vi "AndCriteria.vi"(8 "error in (no error)":errorcluster, 9 "Other Criteria":refnum<class "Criteria.lvclass">, 10 "Criteria":refnum<class "Criteria.lvclass">, 11 "AndCriteria in":refnum<class "AndCriteria.lvclass">) -> (0 "error out":errorcluster, 3 "AndCriteria out":refnum<class "AndCriteria.lvclass">)   [LabVIEW 2018, in "AndCriteria.lvclass"]
uses:
  AndCriteria.lvclass
  Criteria Class/Criteria.lvclass
  AndCriteria.lvclass/AndCriteria.ctl
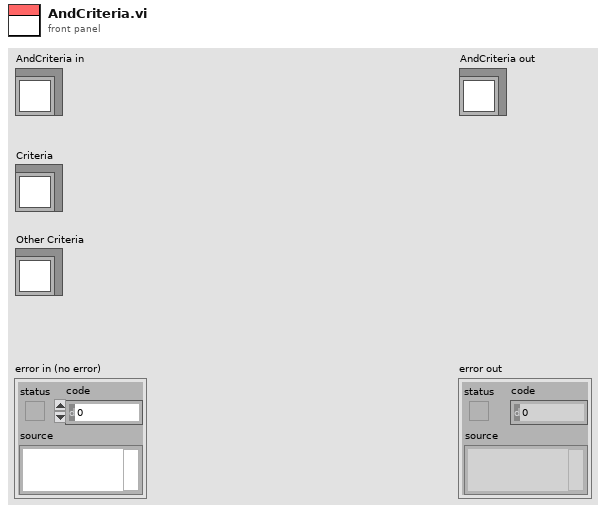
[diagram p1: front panel]
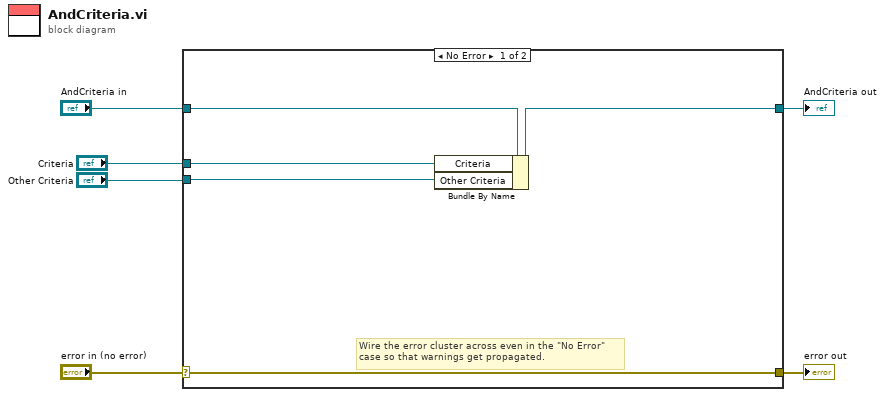
[diagram p0: block diagram]
diagram:
  n1 = case shown="No Error" "error in (no error)" {
    selector: "error in (no error)" -> [w10 w13]
    tunnel: [w10 w13] -> w5
    tunnel: [w9 w12] -> w3
    tunnel: "AndCriteria in" -> [w11 w12]
    tunnel: "Other Criteria" -> [w8 _]
    tunnel: "Criteria" -> [w7 _]
    frame No Error {
      # "Wire the error cluster across even in the \"No Error\"\ncase so that warnings get propagated."
      n2 = Bundle By Name(cluster=w11, "Criteria"=w7, "Other Criteria"=w8) -> (w9:refnum<class "AndCriteria.lvclass">)
    }
    frame Error {
    }
  }
  "error out" <- w5
  "AndCriteria out" <- w3
